vi "labview_ve.vi"() -> ()   [LabVIEW 2020]
uses:
  <vilib>/Utility/file.llb/Read Delimited Spreadsheet (DBL).vi
  <vilib>/Utility/file.llb/Read Delimited Spreadsheet (string).vi
  <vilib>/ptbypt/NI_PtbyPt.lvlib
  <vilib>/gmath/NI_Gmath.lvlib
panel:
  in  "?":enum32{""}(tab)
  out "Entrada":cluster{dbl[], dbl[]}(graph)
  in  "on/off":bool
  in  "Tipo de Onda":u16(ring) items=["Senoidal", "Quadrada", "Genérica"]
  in  "Plot":bool caption="Teste"
  in  "Número de Amostras":dbl
  in  "Amplitude":dbl
  in  "Frequência":dbl
  in  "Fase":dbl
  in  "Taxa de Amostragem":dbl
  in  "Duty Cycle":dbl
  out "Saída":cluster{dbl[], dbl[]}[](graph)
  in  "Importar Arquivos":path=path "C:/Users/Felipe/Desktop/waveform.txt"
  in  "Vc inicial":dbl
  in  "Corrente Inicial":dbl
  in  "R":dbl
  in  "L":dbl
  in  "C":dbl
  in  "Menu Ring":u16(ring) items=["tensão", "corrente", "tensão e corrente", "entrada e saída"]
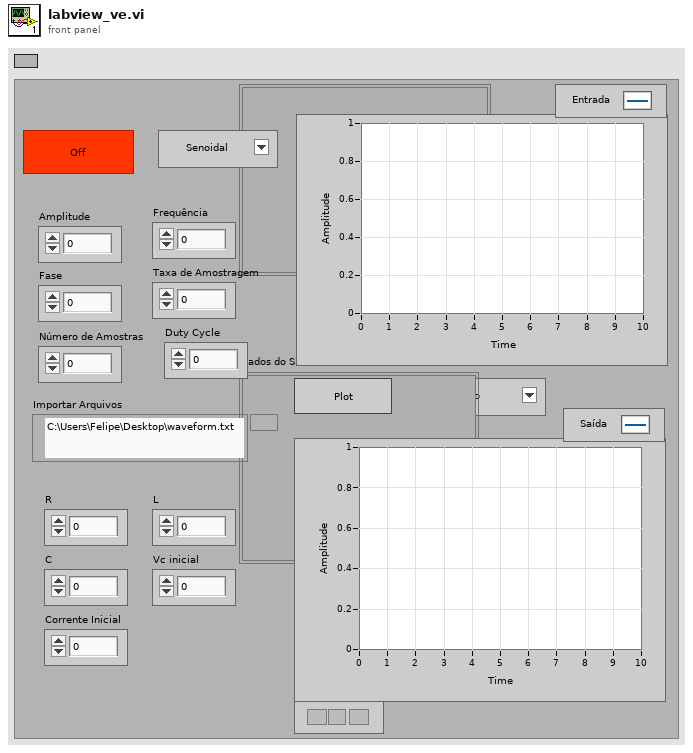
[diagram p1: front panel]
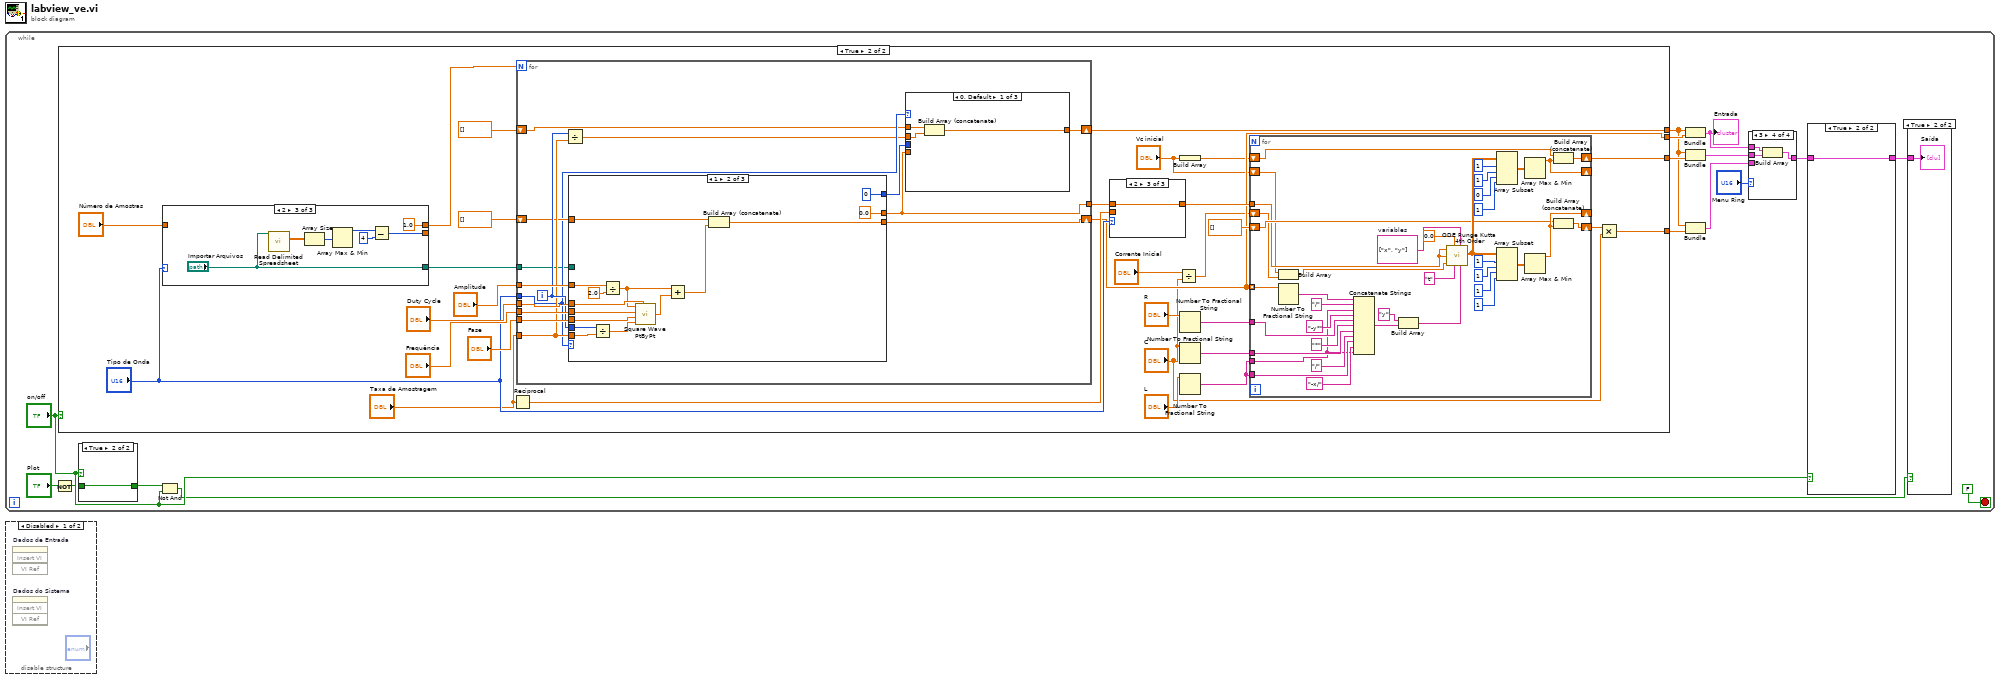
[diagram p0: block diagram]
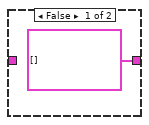
[diagram p2: hidden frame]
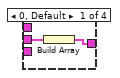
[diagram p5: hidden frame]
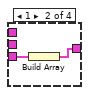
[diagram p6: hidden frame]
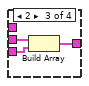
[diagram p7: hidden frame]
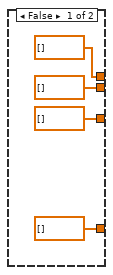
[diagram p8: hidden frame]
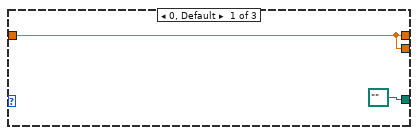
[diagram p11: hidden frame]
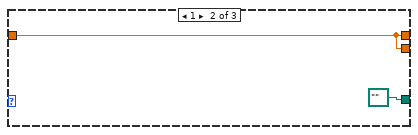
[diagram p12: hidden frame]
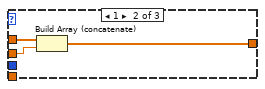
[diagram p13: hidden frame]
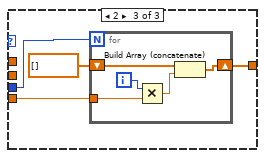
[diagram p14: hidden frame]
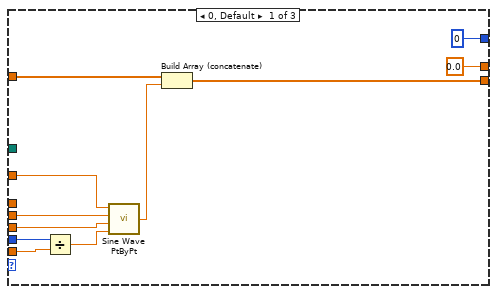
[diagram p15: hidden frame]
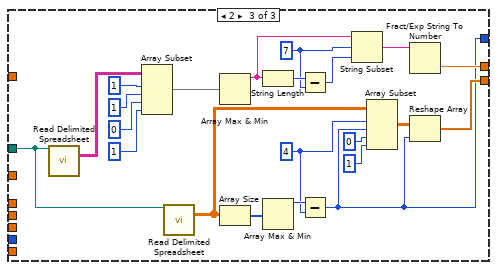
[diagram p16: hidden frame]
diagram:
  n1 = while {
    stop <- FALSE stop-if-true
    n2 = Not(x="Plot") -> (.not. x?=w3:bool)
    n3 = case shown="True" "on/off" {
      tunnel: [dbl[] [] w48] -> w13
      tunnel: [dbl[] [] w47] -> w16
      tunnel: [dbl[] [] w40] -> w15
      tunnel: [dbl[] [] w37] -> w12
      frame False {
      }
      frame True {
        n4 = case shown="2" "Tipo de Onda" {
          tunnel: [w107 w109 1.0 ("Número de Amostras")] -> w59
          tunnel: "Número de Amostras" -> [w107 w109 _]
          tunnel: [path "" ("Importar Arquivos") path "" ("Importar Arquivos") "Importar Arquivos"] -> w57
          tunnel: [w107 w109 w111] -> _
          frame 0, Default {
          }
          frame 1 {
          }
          frame 2 {
            n5 = call-poly <vilib>:"Read Delimited Spreadsheet.vi"("file path (dialog if empty)"="Importar Arquivos") -> ("all rows"=w115:dbl[][])  [unwired: 9 in, 5 out]
            n6 = Array Size(array=w115) -> (size(s)=w117:i32[])
            n7 = Array Max & Min(array=w117) -> (max value=w116:i32)  [unwired: 3 out]
            n8 = Subtract(x=w116, y=4 ("index")) -> (x-y=w111:i32)
          }
        }
        n9 = Reciprocal(x="Taxa de Amostragem") -> (1/x=w49:dbl)
        n10 = for {
          N: w59 -> [_]
          tunnel: "Taxa de Amostragem" -> [w127]
          shift-right: [w121] -> w48
          shift-left: dbl[] [] -> [w123]
          tunnel: "Tipo de Onda" -> [w124]
          tunnel: "Fase" -> [w132]
          tunnel: "Frequência" -> [w131]
          tunnel: "Amplitude" -> [w130]
          shift-right: [w125] -> w47
          shift-left: dbl[] [] -> [w126]
          tunnel: "Duty Cycle" -> [w129]
          tunnel: w57 -> [w119]
          tunnel: [w118] -> w50
          i -> [w128]
          n11 = Divide(x=w128, y=w127) -> (x/y=w122:dbl)
          n12 = case shown="1" w124 {
            tunnel: w132 -> [w156 w170 _]
            tunnel: w131 -> [w155 w171 _]
            tunnel: w130 -> [w154 w162 _]
            tunnel: w128 -> [w152 w172 _]
            tunnel: w129 -> [_ w164 _]
            tunnel: w127 -> [w153 w169 _]
            tunnel: w126 -> [w151 w168 _]
            tunnel: [w150 w167 w177] -> w125
            tunnel: [0.0 0.0 w176] -> w118
            tunnel: [0 0 w175] -> w120
            tunnel: w119 -> [_ _ w174]
            frame 0, Default {
              n13 = Divide(x=w152, y=w153) -> (x/y=w158:dbl)
              n14 = call <vilib>:"Sine Wave PtByPt.vi"("time"=w158, "phase"=w156, "frequency"=w155, "amplitude"=w154) -> ("sine wave"=w157:dbl)
              n15 = Build Array (concatenate)(w151, w157) -> (w150:dbl[])
            }
            frame 1 {
              n16 = Divide(x=w172, y=w169) -> (x/y=w173:dbl)
              n17 = Divide(x=w162, y=2.0) -> (x/y=w161:dbl)
              n18 = call <vilib>:"Square Wave PtByPt.vi"("amplitude"=w161, "frequency"=w171, "phase"=w170, "time"=w173, "duty cycle (%)"=w164) -> ("square wave"=w160:dbl)
              n19 = Add(x=w161, y=w160) -> (x+y=w159:dbl)
              n20 = Build Array (concatenate)(w168, w159) -> (w167:dbl[])
            }
            frame 2 {
              w179 = 4 ("index")
              w187 = 7 ("offset (0)")
              n21 = call-poly <vilib>:"Read Delimited Spreadsheet.vi"("file path (dialog if empty)"=w174) -> ("all rows"=w195:string[][])  [unwired: 9 in, 5 out]
              n22 = Array Subset(array=w195, index (row)=1 ("index"), length (row)=1 ("length"), index (col)=0 ("index"), length (col)=1 ("length")) -> (w190:string[][])
              n23 = call-poly <vilib>:"Read Delimited Spreadsheet.vi"("file path (dialog if empty)"=w174) -> ("all rows"=w180:dbl[][])  [unwired: 9 in, 5 out]
              n24 = Array Max & Min(array=w190) -> (max value=w189:string)  [unwired: 3 out]
              n25 = Array Size(array=w180) -> (size(s)=w184:i32[])
              n26 = String Length(string=w189) -> (length=w188:i32)
              n27 = Array Max & Min(array=w184) -> (max value=w183:i32)  [unwired: 3 out]
              n28 = Subtract(x=w188, y=w187) -> (x-y=w186:i32)
              n29 = Subtract(x=w183, y=w179) -> (x-y=w175:i32)
              n30 = String Subset(string=w189, offset (0)=w187, length (rest)=w186) -> (substring=w185:string)
              n31 = Array Subset(array=w180, index (row)=w179, length (row)=w175, index (col)=0 ("index"), length (col)=1 ("length")) -> (w178:dbl[][])
              n32 = Fract/Exp String To Number(string=w185) -> (number=w176:dbl)  [unwired: 3 in, 1 out]
              n33 = Reshape Array(w178, w175) -> (w177:dbl[])
            }
          }
          n34 = case shown="0, Default" w124 {
            tunnel: w123 -> [w134 w138 _]
            tunnel: w122 -> [w133 w137 _]
            tunnel: [w135 w136 w139] -> w121
            tunnel: w118 -> [_ _ w141]
            tunnel: w120 -> [_ _ w142]
            frame 0, Default {
              n35 = Build Array (concatenate)(w134, w133) -> (w135:dbl[])
            }
            frame 1 {
              n36 = Build Array (concatenate)(w138, w137) -> (w136:dbl[])
            }
            frame 2 {
              n37 = for {
                N: w142 -> [_]
                tunnel: w141 -> [w147]
                shift-right: [w144] -> w139
                shift-left: dbl[] [] -> [w143]
                i -> [w146]
                n38 = Multiply(x=w146, y=w147) -> (x*y=w145:dbl)
                n39 = Build Array (concatenate)(w143, w145) -> (w144:dbl[])
              }
            }
          }
        }
        n40 = case shown="2" "Tipo de Onda" {
          tunnel: [w66 w67 w68] -> w51
          tunnel: w50 -> [_ _ w68]
          tunnel: w49 -> [w66 w67 _]
          frame 0, Default {
          }
          frame 1 {
          }
          frame 2 {
          }
        }
        n41 = Divide(x="Corrente Inicial", y="C") -> (x/y=w43:dbl)
        n42 = Build Array("Vc inicial") -> (w41:dbl[])
        n43 = Number To Fractional String(number="R") -> (F-format string=w56:string)  [unwired: 3 in]
        n44 = Number To Fractional String(number="C") -> (F-format string=w55:string)  [unwired: 3 in]
        n45 = Number To Fractional String(number="L") -> (F-format string=w54:string)  [unwired: 3 in]
        n46 = for {
          tunnel: w47 -> [w106] mode=indexing
          tunnel: w54 -> [w90]
          tunnel: w56 -> [w96]
          tunnel: w55 -> [w94]
          tunnel: w54 -> [w92]
          shift-right: [w85] -> _
          shift-left: w43 -> [w69]
          shift-right: [w83] -> _
          shift-left: "Vc inicial" -> [w70]
          shift-right: [w82] -> w39
          shift-left: dbl[] [] ("array") -> [w84]
          tunnel: w51 -> [w73]
          shift-right: [w71] -> w40
          shift-left: w41 -> [w72]
          w100 = string[] ["x", "y"]  # variables
          n47 = Build Array(w70, w69) -> (w102:dbl[])
          n48 = Number To Fractional String(number=w106) -> (F-format string=w99:string)  [unwired: 3 in]
          n49 = Concatenate Strings(w99, "/" ("string"), w90, "-y*" ("string"), w96, "*" ("string"), w94, "/" ("string"), w92, "-x/" ("string"), w90) -> (w89:string)
          n50 = Build Array("y", w89) -> (w104:string[])
          n51 = call <vilib>:"ODE Runge Kutta 4th Order.vi"("time end"=w73, "time start"=0.0, "h (step rate)"=w73, "X0"=w102, "time"="t", "X (name of variables)"=w100, "F(X,t) (right sides of the ODE\nas functions of X and t)"=w104) -> ("X Values (solution)"=w88:dbl[][])  [unwired: 3 out]
          n52 = Array Subset(array=w88, index (row)=1 ("index"), length (row)=1 ("length"), index (col)=0 ("index"), length (col)=1 ("length")) -> (w86:dbl[][])
          n53 = Array Subset(array=w88, index (row)=1 ("index"), length (row)=1 ("length"), index (col)=1 ("index"), length (col)=1 ("length")) -> (w87:dbl[][])
          n54 = Array Max & Min(array=w86) -> (max value=w83:dbl)  [unwired: 3 out]
          n55 = Array Max & Min(array=w87) -> (max value=w85:dbl)  [unwired: 3 out]
          n56 = Build Array (concatenate)(w72, w83) -> (w71:dbl[])
          n57 = Build Array (concatenate)(w84, w85) -> (w82:dbl[])
        }
        n58 = Multiply(x=w39, y="C") -> (x*y=w37:dbl[])
      }
    }
    n59 = case shown="True" "on/off" {
      selector: "on/off" -> [w19 _]
      tunnel: [w19 w20] -> w6
      tunnel: w3 -> [_ w20]
      frame False {
      }
      frame True {
      }
    }
    n60 = Not And(1:"on/off", 2:w6) -> (0:w5:bool)
    n61 = Bundle(w13, w16) -> (w1:cluster{dbl[], dbl[]})  [unwired: 1 in]
    "Entrada" <- w1
    n62 = Bundle(w13, w15) -> (w11:cluster{dbl[], dbl[]})  [unwired: 1 in]
    n63 = Bundle(w13, w12) -> (w10:cluster{dbl[], dbl[]})  [unwired: 1 in]
    n64 = case shown="3" "Menu Ring" {
      tunnel: w11 -> [w23 _ w26 w30]
      tunnel: [w22 w24 w28 w29] -> w8
      tunnel: w10 -> [_ w25 w27 _]
      tunnel: w1 -> [_ _ _ w31]
      frame 0, Default {
        n65 = Build Array(w23) -> (w22:cluster{dbl[], dbl[]}[])
      }
      frame 1 {
        n66 = Build Array(w25) -> (w24:cluster{dbl[], dbl[]}[])
      }
      frame 2 {
        n67 = Build Array(w26, w27) -> (w28:cluster{dbl[], dbl[]}[])
      }
      frame 3 {
        n68 = Build Array(w31, w30) -> (w29:cluster{dbl[], dbl[]}[])
      }
    }
    n69 = case shown="True" "on/off" {
      tunnel: [cluster{dbl[], dbl[]}[] [] w18] -> w9
      tunnel: w8 -> [_ w18]
      frame False {
      }
      frame True {
      }
    }
    n70 = case shown="True" w5 {
      tunnel: w9 -> [_ w21]
      frame False {
      }
      frame True {
        "Saída" <- w21
      }
    }
  }
  n71 = disable-structure shown="Disabled" {
    frame Disabled {
      n72 = invoke on="Dados de Entrada" class="SubPnl" method="Insert VI"() -> ()  [unwired: 4 in, 4 out]
      n73 = invoke on="Dados do Sistema" class="SubPnl" method="Insert VI"() -> ()  [unwired: 4 in, 4 out]
    }
    frame Enabled {
    }
  }
